vi "XIPIN_Ethernet_PHY_MII_to_Reduced_MII_2_0.vi"   [LabVIEW 2017]
doc: "MII to RMII provides the RMII between RMII-compliant ethernet physical media devices and XPS Ethernet Lite.\n------------------------------------\n<b>Need License</b> : No"
uses:
  <vilib>/rvi/XilinxIP/XIPIN_XNode/niFpgaXIPIN.xnode
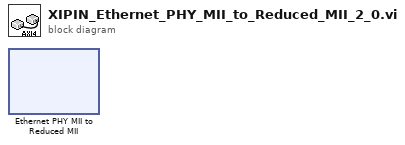
[diagram p0: block diagram]
diagram:
  n1 = xnode ("Ethernet PHY MII to Reduced MII")() -> ()
